vi "SR630_subvi.vi"(10 "Write Buffer":string, 11 "VISA Refnum in":refnum<visa-resource-name>) -> (3 "read buffer":string)   [LabVIEW 2013]
uses:
  <vilib>/Instr/_visa.llb/VISA Open Access Mode.ctl
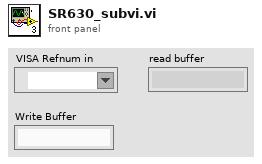
[diagram p1: front panel]
types:
  T1 = typedef "VISA Open Access Mode.ctl" = u32
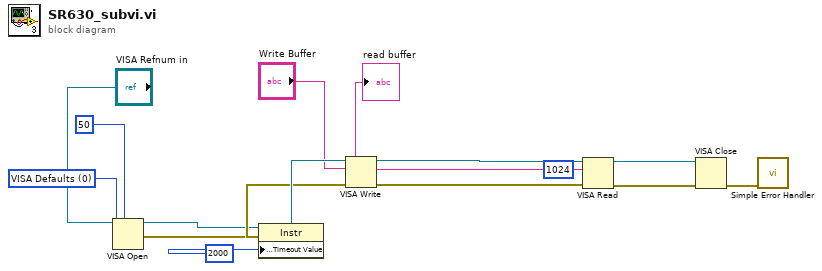
[diagram p0: block diagram]
diagram:
  w10 = T1 0 items=["VISA Defaults"=0, "Exclusive Lock"=1, "Load Configured Settings"=4] ("Access Mode")
  n1 = VISA Open(timeout (0)=u32 50 ("VISA Open timeout (0)"), access mode=w10, VISA resource name="VISA Refnum in") -> (VISA resource name=w7:refnum<visa-resource-name>, error out=w8:errorcluster)  [unwired: 2 in]
  n2 = property class="Instr"(reference=w7, error in=w8, "General Settings:Timeout Value"=u32 2000) -> (reference out=w16:refnum<visa-resource-name>, error out=w15:errorcluster)
  n3 = VISA Write(VISA resource name=w16, write buffer="Write Buffer", error in (no error)=w15) -> (VISA resource name out=w1:refnum<visa-resource-name>, error out=w3:errorcluster)  [unwired: 1 out]
  n4 = VISA Read(VISA resource name=w1, byte count=u32 1024, error in (no error)=w3) -> (VISA resource name out=w2:refnum<visa-resource-name>, read buffer=→"read buffer":string, error out=w4:errorcluster)  [unwired: 1 out]
  n5 = VISA Close(VISA resource name=w2, error in (no error)=w4) -> (error out=w13:errorcluster)
  n6 = call <vilib>:"Simple Error Handler.vi"("error in (no error)"=w13) -> ()  [unwired: 4 in, 5 out]
